vi "Sequence.Test.Unload.vi"(7 "Code in":T1={"Ready"=FALSE, "DoubleOrder"=FALSE, "OrderDone"=FALSE, "AllowSingleSlot"=FALSE, "TunedA"=FALSE, "TunedB"=FALSE, "CheckDM"=FALSE, "ThresholdA"=0, "ThresholdB"=0, "Plate"=enum."Wabco", "ImgPath"=path "", "Variant"={"State"=enum."Init", "ImgPath"=path "", "WabcoPlate"="", "WabcoProduct"="", "ClientProduct"="", "ClientPlate"="", "TotalQuantity"=0, "OrderQuantity"=0, "Serial"=0, "Wabco"={"LaserJob"="", "AdditionalTxt"="037", "FactoryCode"="", "RevID"=0, "ForkID"=0, "FailuresLimit"=0, "GlobalCnt"=0, "Bank"=0, "SerialFormat"=enum."6 dig", "CoordA"={"X"=0.0, "Y"=0.0, "Angle"=0.0}, "CoordB"={"X"=0.0, "Y"=0.0, "Angle"=0.0}, "DMCconfig"=0}, "Client"={"LaserJob"="", "AdditionalTxt"="", "FactoryCode"="037", "RevID"=0, "ForkID"=0, "FailuresLimit"=0, "GlobalCnt"=0, "Bank"=0, "SerialFormat"=enum."6 dig", "CoordA"={"X"=0.0, "Y"=0.0, "Angle"=0.0}, "CoordB"={"X"=0.0, "Y"=0.0, "Angle"=0.0}, "DMCconfig"=0}}}, 8 "error in":errorcluster, 11 "Data in":T8) -> (0 "error out":errorcluster, 3 "Data out":T8)   [LabVIEW 2016]
uses:
  Sequence.Test.Status.ctl
  Sequence.Slot.StatusData.ctl
  Sequence.Test.Unload.Status.ctl
  Sequence.Prod.StatusData.ctl
  Sequence.Step.Status.ctl
  Sequence.Test.BreakReason.ctl
  Sequence.Code.Sets.ctl
  Sequence.PlateType.ctl
  Logger/Logger.Variant.Sets.ctl
  Station/Station.Changeover.State.vi
  Station/Station.Plate.Properties.ctl
  Sequence.Code.SerialFormat.ctl
  Drivers/V7310/LowLevel/V7310.Job.Sets.ctl
  Drivers/FestoCPX/Station/FestoCPX.Station.ProdArmPosition.ctl
  Station/Station.ProductSlot.ctl
  Station/Station.ValvePosition.ctl
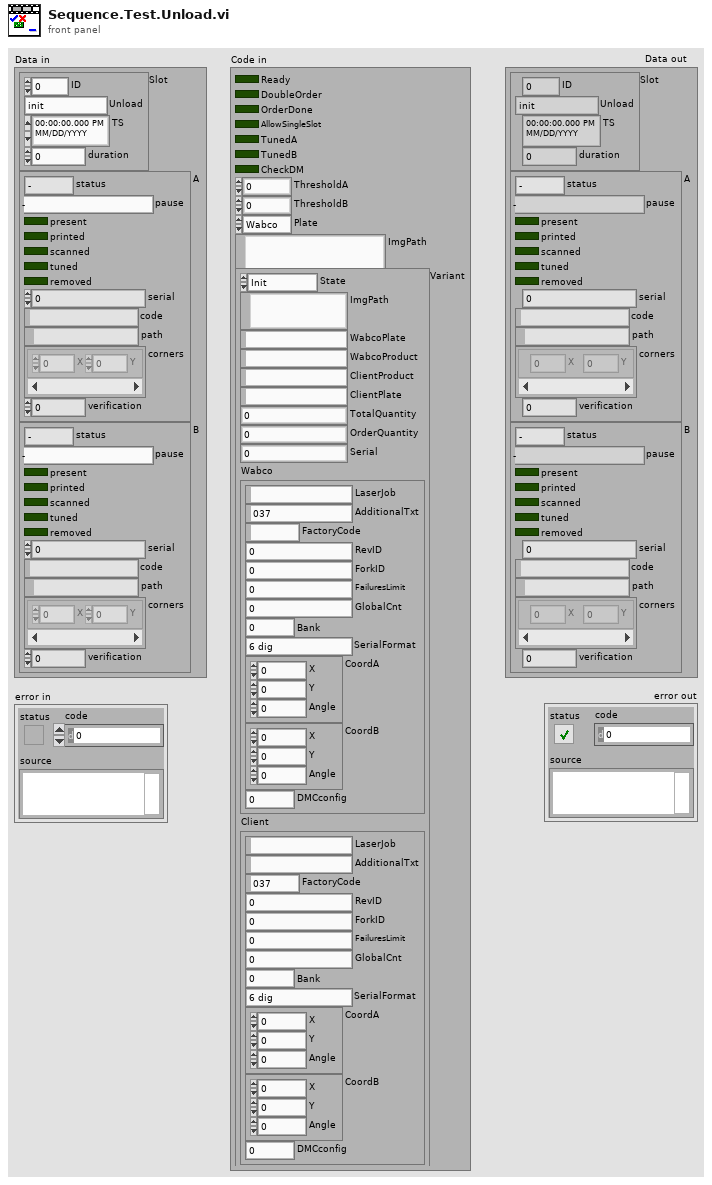
[diagram p1: front panel]
types:
  T1 = typedef "Sequence.Code.Sets.ctl" = cluster{"Ready":bool, "DoubleOrder":bool, "OrderDone":bool, "AllowSingleSlot":bool, "TunedA":bool, "TunedB":bool, "CheckDM":bool, "ThresholdA":u8, "ThresholdB":u8, "Plate":T2, "ImgPath":path, "Variant":T3}
  T2 = typedef "Sequence.PlateType.ctl" = enum16{"Wabco", "Client"}
  T3 = typedef "Logger.Variant.Sets.ctl" = cluster{"State":T4, "ImgPath":path, "WabcoPlate":string, "WabcoProduct":string, "ClientProduct":string, "ClientPlate":string, "TotalQuantity":u16, "OrderQuantity":u16, "Serial":i32, "Wabco":T5, "Client":T5}
  T4 = typedef "Station.Changeover.State.vi" = enum16{"Init", "Scaning", "NOK", "Wait for ack", "Ready"}
  T5 = typedef "Station.Plate.Properties.ctl" = cluster{"LaserJob":string, "AdditionalTxt":string, "FactoryCode":string, "RevID":u8, "ForkID":u8, "FailuresLimit":u16, "GlobalCnt":i32, "Bank":u8, "SerialFormat":T6, "CoordA":T7, "CoordB":T7, "DMCconfig":i32}
  T6 = typedef "Sequence.Code.SerialFormat.ctl" = enum8{"", "6 dig", "7 dig"}
  T7 = typedef "V7310.Job.Sets.ctl" = cluster{"X":dbl, "Y":dbl, "Angle":dbl}
  T8 = typedef "Sequence.Test.Status.ctl" = cluster{"Slot":T9, "A":T11, "B":T11}
  T9 = typedef "Sequence.Slot.StatusData.ctl" = cluster{"ID":i32, "Unload":T10, "TS":timestamp, "duration":u32}
  T10 = typedef "Sequence.Test.Unload.Status.ctl" = enum16{"init", "check NOK", "check OK", "wait on NOK", "wait on OK", "wait on Unload", "done"}
  T11 = typedef "Sequence.Prod.StatusData.ctl" = cluster{"status":T12, "pause":T13, "present":bool, "printed":bool, "scanned":bool, "tuned":bool, "removed":bool, "serial":i32, "code":string, "path":path, "corners":cluster{"X":i32, "Y":i32}[], "verification":u8}
  T12 = typedef "Sequence.Step.Status.ctl" = enum16{"-", "Pending", "Running", "Skipped", "Passed", "Failed", "Done", "Error", "Aborted", "Stopped"}
  T13 = typedef "Sequence.Test.BreakReason.ctl" = enum16{"-", "NOK container", "OK container", "Rev empty", "Rev missing", "Rev wrong", "Fork missing", "Fork wrong", "NOK limit", "Unload failure", "Single slot", "Part done", "Err: Prod move work", "Err: Prod move home", "Err: Prod lift work", "Err: Prod lift home", "Err: Prod Arm Work", "Err: Prod Arm NOK", "Err: Prod Arm OK", "Err: Prod NOK suck", "Err: Prod NOK drop", "Err: Prod OK missing", "Err: Prod OK suck", "Err: Prod OK drop"}
  T14 = typedef "FestoCPX.Station.ProdArmPosition.ctl" = enum16{"Work", "OK", "NOK"}
  T15 = typedef "Station.ProductSlot.ctl" = enum8{"A", "B"}
  T16 = typedef "FestoCPX.Station.ProdPresent.ctl" = cluster{"Slot1":cluster{"A":bool, "B":bool}, "Slot2":cluster{"A":bool, "B":bool}, "Slot3":cluster{"A":bool, "B":bool}, "Slot4":cluster{"A":bool, "B":bool}, "Final":cluster{"A":bool, "B":bool}, "OK":cluster{"A":bool, "B":bool}, "Container":cluster{"OK":bool, "NOK":bool}}
  T17 = typedef "Station.ValvePosition.ctl" = enum16{"Home", "Work"}
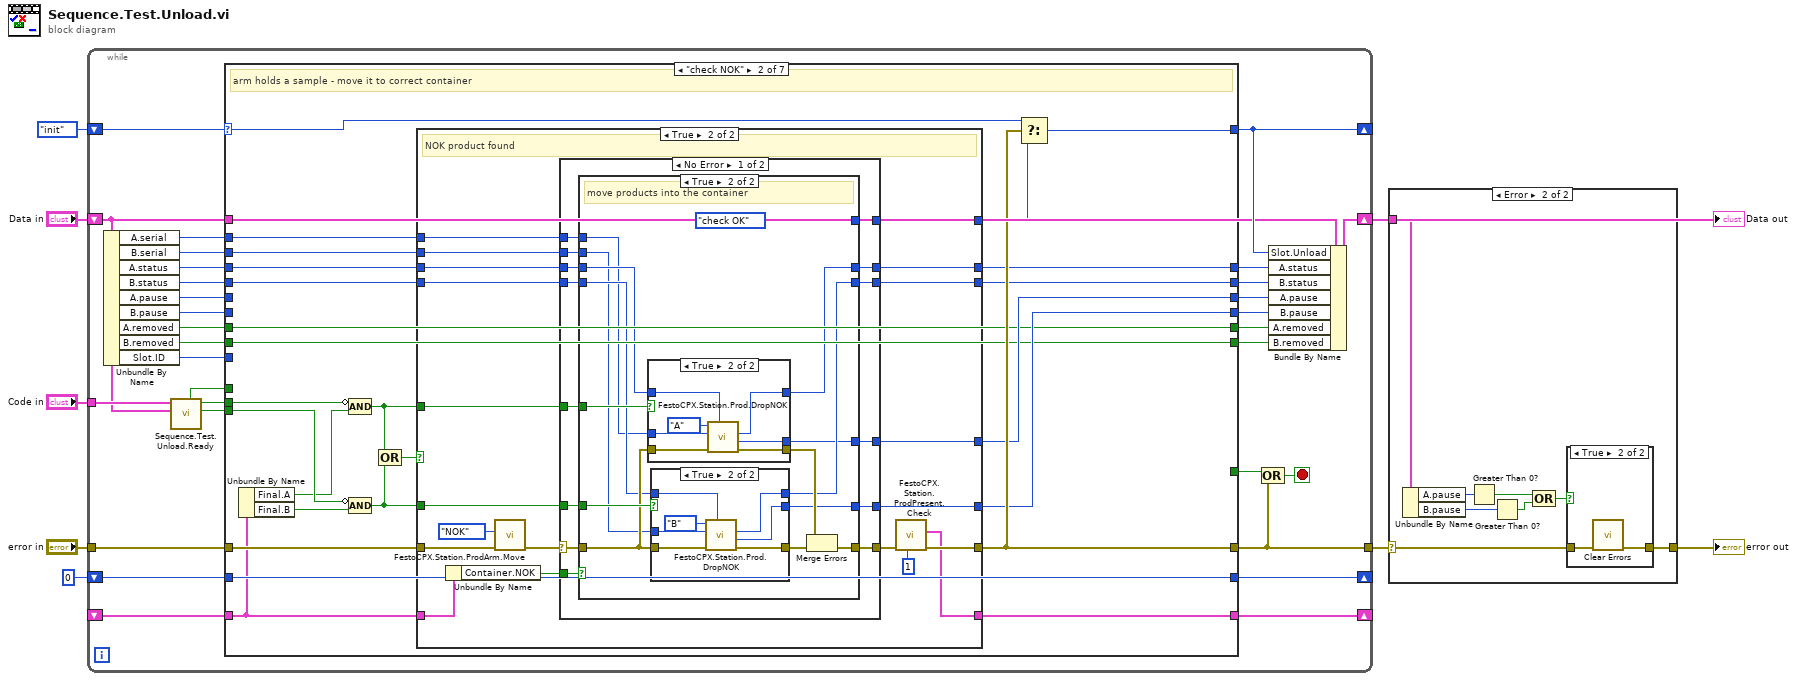
[diagram p0: block diagram]
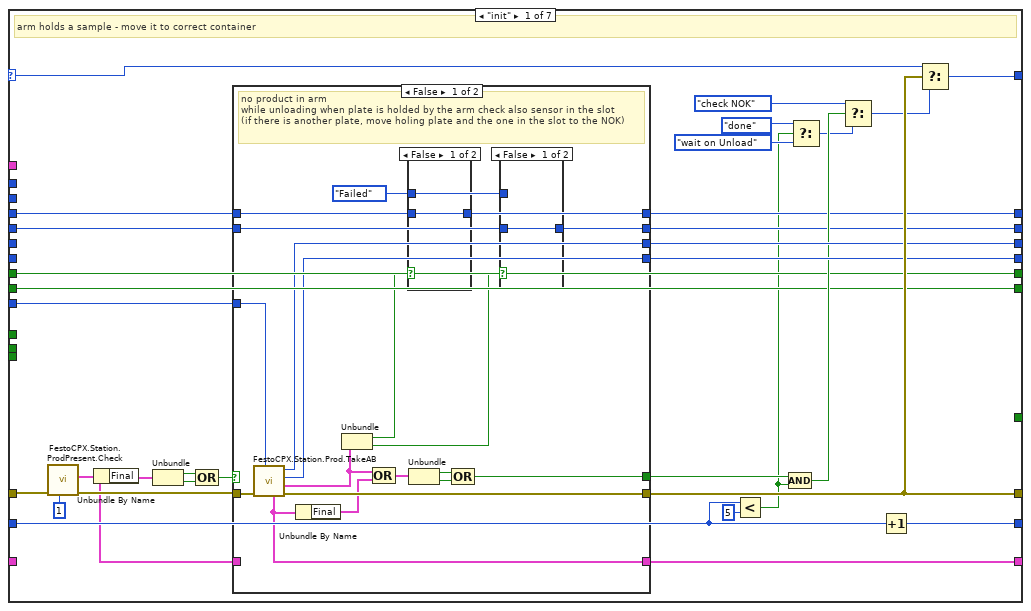
[diagram p2: hidden frame]
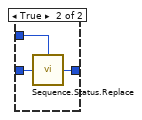
[diagram p3: hidden frame]
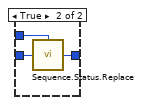
[diagram p4: hidden frame]
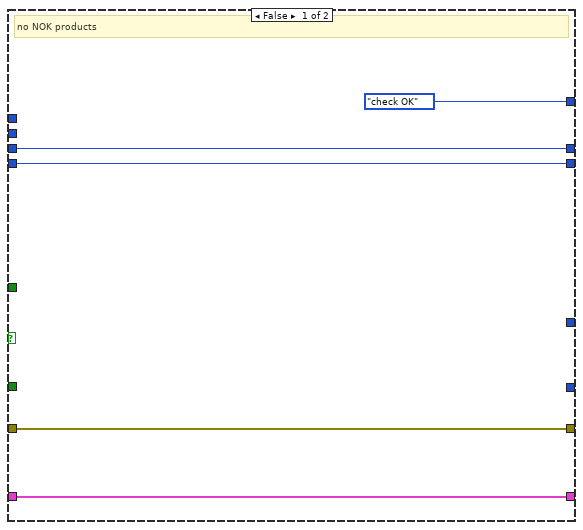
[diagram p6: hidden frame]
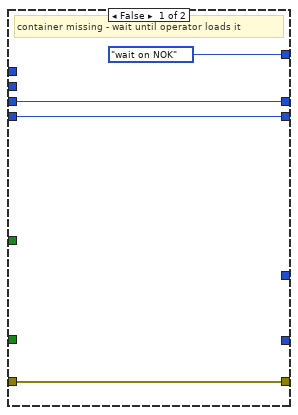
[diagram p7: hidden frame]
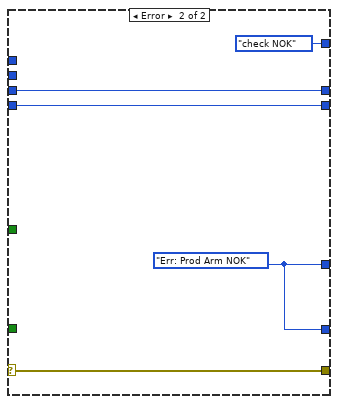
[diagram p10: hidden frame]
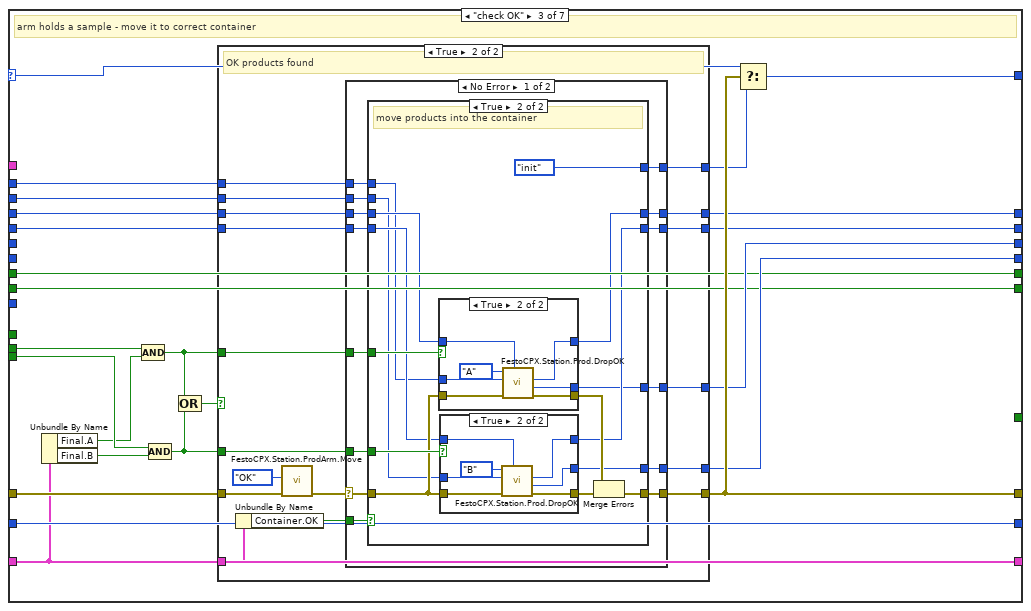
[diagram p11: hidden frame]
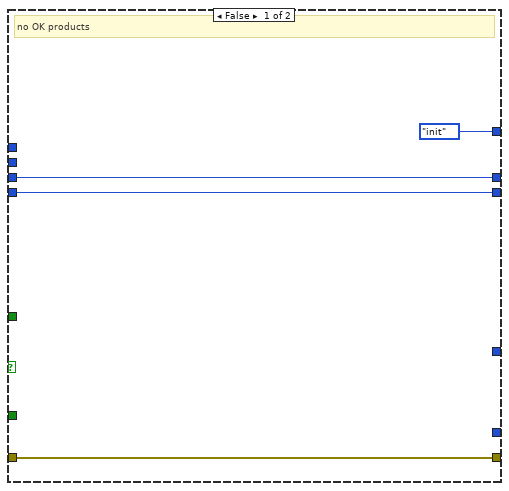
[diagram p12: hidden frame]
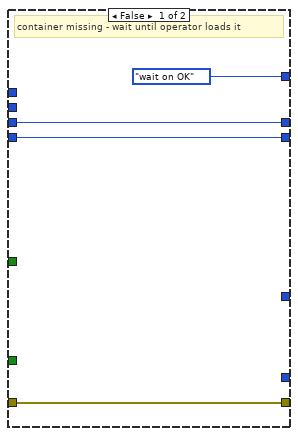
[diagram p13: hidden frame]
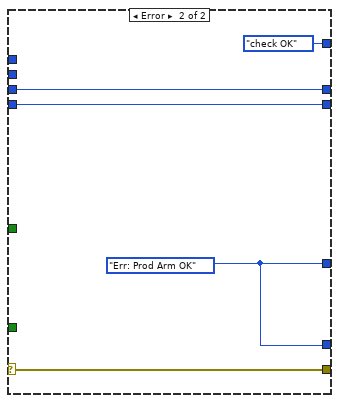
[diagram p16: hidden frame]
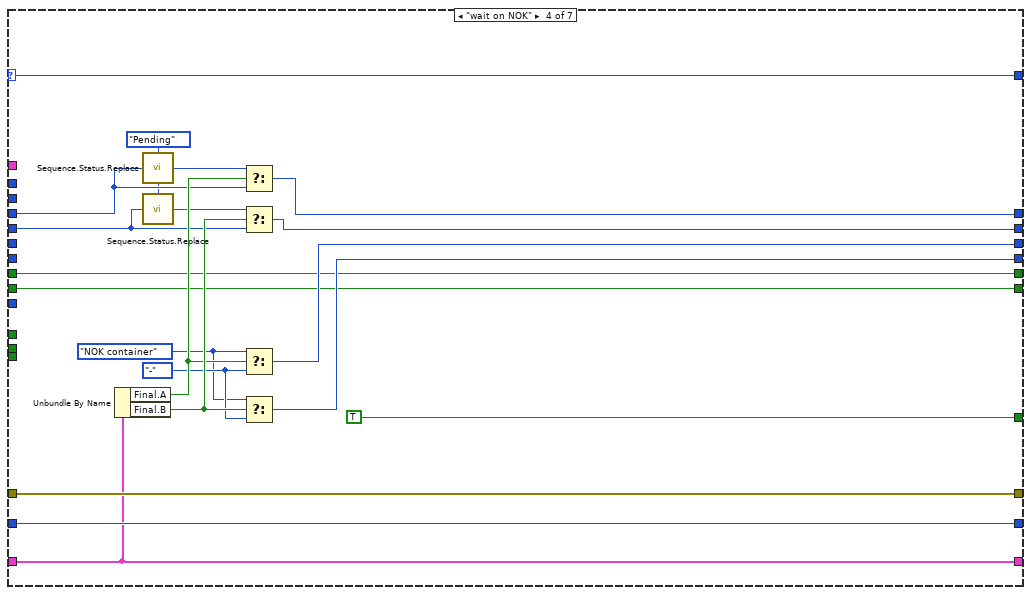
[diagram p17: hidden frame]
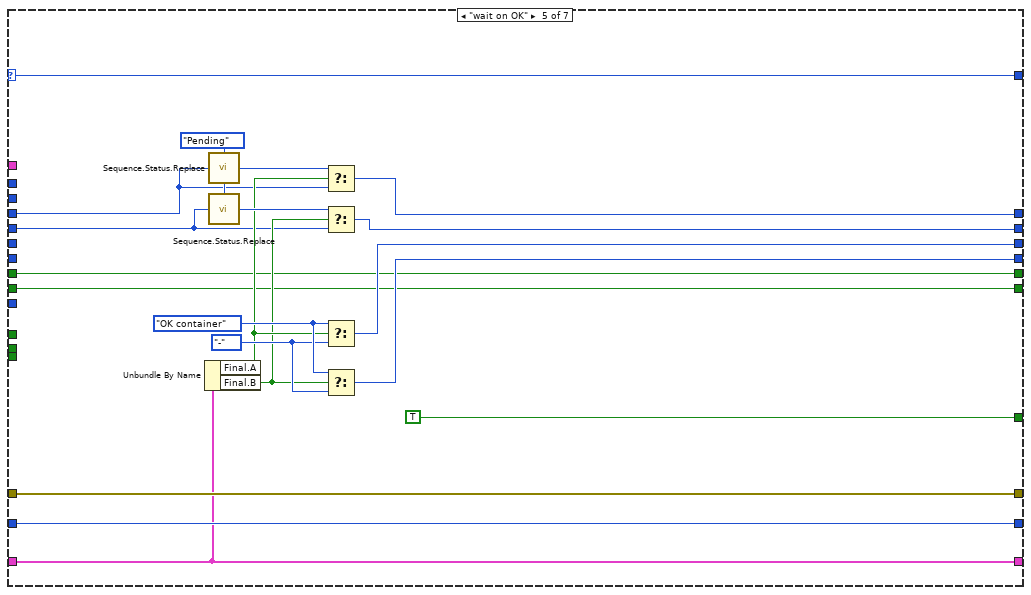
[diagram p18: hidden frame]
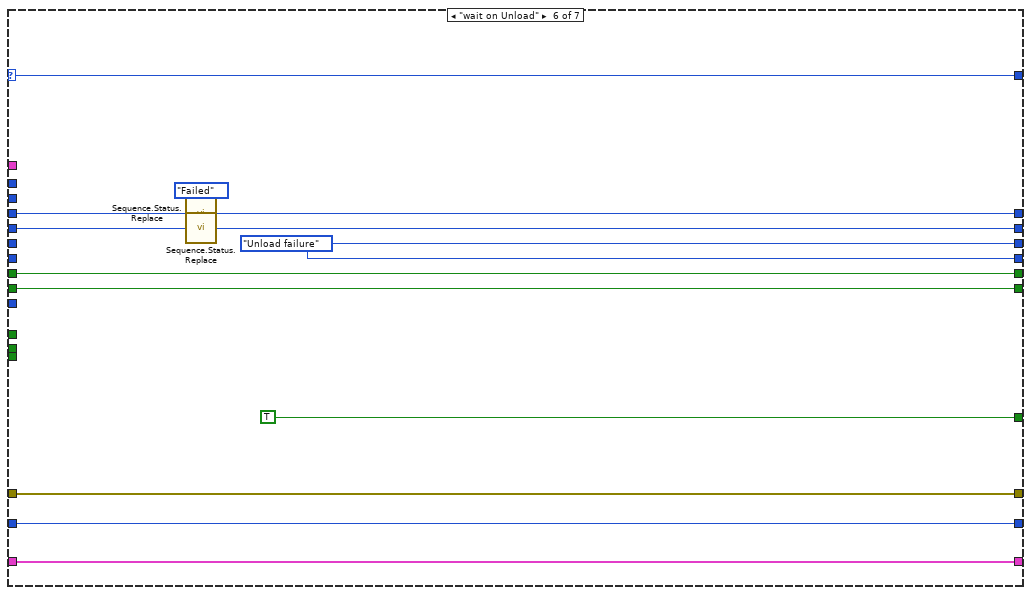
[diagram p19: hidden frame]
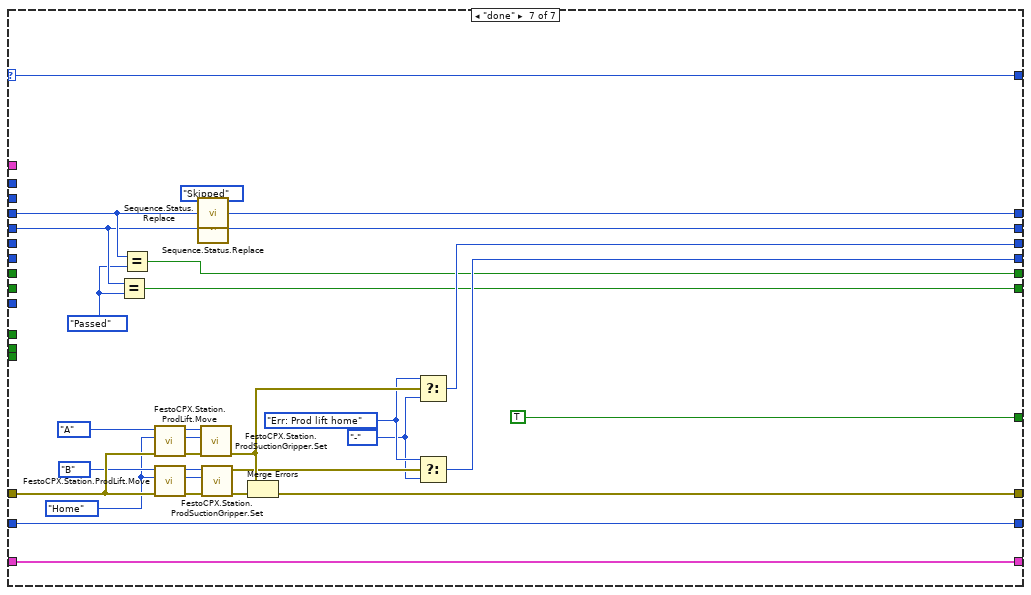
[diagram p20: hidden frame]
diagram:
  n1 = while {
    shift-right: [w34] -> w1
    shift-left: "Data in" -> [w25]
    tunnel: "error in" -> [w15]
    tunnel: [w37] -> w3
    shift-right: [w33] -> _
    shift-left: Sequence.Test.Unload.Status."init" ("Slot.Unload") -> [w36]
    tunnel: "Code in" -> [w26]
    shift-right: [w21] -> _
    shift-left: 0 -> [w22]
    shift-right: [w14] -> _
    shift-left: _ -> [w13]
    stop <- w39 stop-if-true
    n2 = Unbundle By Name(w25) -> ("A.serial"=w28:i32, "B.serial"=w27:i32, "A.status"=w31:T12, "B.status"=w32:T12, "A.pause"=w18:T13, "B.pause"=w17:T13, "A.removed"=w12:bool, "B.removed"=w11:bool, "Slot.ID"=w35:i32)
    n3 = call "Sequence.Test.Unload.Ready.vi"("Data in"=w25, "Code"=w26) -> ("OK B"=w23:bool, "OK A"=w24:bool, "PartialOrder"=w16:bool)  [unwired: 7 in]
    n4 = case shown="\"check NOK\"" w36 {
      selector: w36 -> [w66 w121 w227 w330 w350 w363 w382]
      tunnel: w15 -> [w55 w125 w216 w328 w348 w361 w387]
      tunnel: [w71 w128 w233 w328 w348 w361 w381] -> w37
      tunnel: [_ _ _ TRUE TRUE TRUE TRUE] -> w38
      tunnel: [w70 w126 w231 w330 w350 w363 w382] -> w33
      tunnel: w35 -> [w51 _ _ _ _ _ _]
      tunnel: w25 -> [_ _ _ _ _ _ _]
      tunnel: w32 -> [w47 w118 w223 w316 w337 w356 w366]
      tunnel: w31 -> [w49 w120 w224 w315 w336 w359 w368]
      tunnel: [w46 w117 w226 w322 w335 w357 w379] -> w30
      tunnel: [w48 w119 w225 w323 w334 w358 w380] -> w29
      tunnel: [w64 w113 w217 w327 w347 w354 w371] -> w20
      tunnel: [w63 w112 w212 w326 w346 w354 w370] -> w19
      tunnel: w28 -> [_ w116 w222 _ _ _ _]
      tunnel: w27 -> [_ w115 w221 _ _ _ _]
      tunnel: w24 -> [_ w111 w219 _ _ _ _]
      tunnel: w23 -> [_ w110 w220 _ _ _ _]
      tunnel: w22 -> [w58 w114 w218 w321 w345 w360 w377]
      tunnel: [w65 w114 w218 w321 w345 w360 w377] -> w21
      tunnel: w18 -> [_ _ _ _ _ _ _]
      tunnel: w17 -> [_ _ _ _ _ _ _]
      tunnel: w16 -> [_ _ _ _ _ _ _]
      tunnel: [w62 w109 w213 w313 w333 w353 w369] -> w14
      tunnel: w13 -> [_ w108 w213 w313 w333 w353 w369]
      tunnel: w12 -> [w45 w105 w211 w312 w332 w352 _]
      tunnel: w11 -> [w44 w104 w210 w311 w331 w351 _]
      tunnel: [w45 w105 w211 w312 w332 w352 w367] -> w10
      tunnel: [w44 w104 w210 w311 w331 w351 w364] -> w9
      frame "init" {
        # "arm holds a sample - move it to correct container"
        n5 = call "FestoCPX.Station.ProdPresent.Check.vi"("Stab Counter (0)"=1 ("Max Stab time [ms] (0)"), "error in"=w55) -> ("error out"=w54:errorcluster, "Prod Present"=w52:T16)  [unwired: 4 in, 4 out]
        n6 = Unbundle By Name(w52) -> ("Final"=w53:cluster{"A":bool, "B":bool})
        n7 = Unbundle(w53) -> ("A"=w69:bool, "B"=w68:bool)
        n8 = Compound Arithmetic op=OR(w69, w68) -> (w67:bool)
        n9 = case shown="False" w67 {
          selector: w67 -> [_ w101]
          tunnel: [w80 w103] -> w71
          tunnel: w54 -> [w90 w103]
          tunnel: [w89 _] -> w64
          tunnel: [w88 _] -> w63
          tunnel: [w79 w102] -> w62
          tunnel: w52 -> [_ w102]
          tunnel: [w75 w101] -> w57
          tunnel: w51 -> [w87 _]
          tunnel: w49 -> [w86 w100]
          tunnel: [w83 w100] -> w48
          tunnel: w47 -> [w84 w99]
          tunnel: [w82 w99] -> w46
          frame False {
            w85 = Sequence.Step.Status."Failed" ("t")
            # "no product in arm\nwhile unloading when plate is holded by the arm check also sensor in the slot \n(if there is another plate, move holing plate and the one in the slot to the NOK)"
            n10 = call "FestoCPX.Station.Prod.TakeAB.vi"("SuckerID"=w87, "error in"=w90) -> ("error out"=w80:errorcluster, "Slot"=w73:cluster{"A":bool, "B":bool}, "Error reason B"=w88:T13, "Error reason A"=w89:T13, "Prod Present"=w79:T16)  [unwired: 5 in]
            n11 = Unbundle By Name(w79) -> ("Final"=w72:cluster{"A":bool, "B":bool})
            n12 = Unbundle(w73) -> ("A"=w74:bool, "B"=w81:bool)
            n13 = Compound Arithmetic op=OR(w73, w72) -> (w78:cluster{"A":bool, "B":bool})
            n14 = case shown="False" w74 {
              tunnel: w86 -> [w95 w98]
              tunnel: w85 -> [_ w97]
              tunnel: [w95 w96] -> w83
              frame False {
              }
              frame True {
                n15 = call "Sequence.Status.Replace.vi"("old status"=w98, "new status (Done)"=w97) -> ("status out"=w96:T12)
              }
            }
            n16 = Unbundle(w78) -> ("A"=w77:bool, "B"=w76:bool)
            n17 = Compound Arithmetic op=OR(w77, w76) -> (w75:bool)
            n18 = case shown="False" w81 {
              tunnel: w84 -> [w91 w94]
              tunnel: w85 -> [_ w93]
              tunnel: [w91 w92] -> w82
              frame False {
              }
              frame True {
                n19 = call "Sequence.Status.Replace.vi"("old status"=w94, "new status (Done)"=w93) -> ("status out"=w92:T12)
              }
            }
          }
          frame True {
            # "arm already holds product"
          }
        }
        n20 = Less?(x=w58, y=5) -> (x < y?=w41:bool)
        n21 = Compound Arithmetic op=AND(w57, w41) -> (w56:bool)
        n22 = Select(t=Sequence.Test.Unload.Status."done" ("Slot.Unload"), s=w41, f=Sequence.Test.Unload.Status."wait on Unload" ("Slot.Unload")) -> (s? t:f=w40:T10)
        n23 = Select(t=Sequence.Test.Unload.Status."check NOK" ("Slot.Unload"), s=w56, f=w40) -> (s? t:f=w59:T10)
        n24 = Increment(x=w58) -> (x+1=w65:i32)
        n25 = Select(t=w66, s=w71, f=w59) -> (s? t:f=w70:T10)
      }
      frame "check NOK" {
        # "arm holds a sample - move it to correct container"
        n26 = Unbundle By Name(w108) -> ("Final.A"=w107:bool, "Final.B"=w106:bool)
        n27 = Compound Arithmetic op=AND(invert w111, w107) -> (w123:bool)
        n28 = Compound Arithmetic op=AND(invert w110, w106) -> (w122:bool)
        n29 = Compound Arithmetic op=OR(w123, w122) -> (w124:bool)
        n30 = case shown="True" w124 {
          tunnel: w123 -> [_ w153]
          tunnel: w122 -> [_ w152]
          tunnel: w125 -> [w132 w150]
          tunnel: [w132 w136] -> w128
          tunnel: [Sequence.Test.Unload.Status."check OK" ("Slot.Unload") w149] -> w127
          tunnel: w120 -> [w131 w148]
          tunnel: [w131 w147] -> w119
          tunnel: w118 -> [w130 w146]
          tunnel: [w130 w145] -> w117
          tunnel: w116 -> [_ w144]
          tunnel: w115 -> [_ w143]
          tunnel: [_ w141] -> w113
          tunnel: [_ w140] -> w112
          tunnel: [w129 w135] -> w109
          tunnel: w108 -> [w129 w139]
          frame False {
            # "no NOK products"
          }
          frame True {
            # "NOK product found"
            n31 = Unbundle By Name(w139) -> ("Container.NOK"=w142:bool)
            n32 = call "FestoCPX.Station.ProdArm.Move.vi"("error in"=w150, "Product Status"=FestoCPX.Station.ProdArmPosition."NOK") -> ("error out"=w138:errorcluster)  [unwired: 9 in]
            n33 = case shown="No Error" w138 {
              selector: w138 -> [w154 w209]
              tunnel: w153 -> [w167 _]
              tunnel: w152 -> [w166 _]
              tunnel: [w165 w209] -> w137
              tunnel: [w164 Sequence.Test.Unload.Status."check NOK" ("Slot.Unload")] -> w149
              tunnel: w148 -> [w163 w208]
              tunnel: [w162 w208] -> w147
              tunnel: w146 -> [w161 w207]
              tunnel: [w160 w207] -> w145
              tunnel: w144 -> [w159 _]
              tunnel: w143 -> [w158 _]
              tunnel: w142 -> [w157 _]
              tunnel: [w156 w206] -> w141
              tunnel: [w155 w206] -> w140
              frame No Error {
                n34 = case shown="True" w157 {
                  tunnel: w167 -> [_ w186]
                  tunnel: w166 -> [_ w185]
                  tunnel: [w170 w182] -> w165
                  tunnel: w154 -> [w170 w181]
                  tunnel: [Sequence.Test.Unload.Status."wait on NOK" ("Slot.Unload") Sequence.Test.Unload.Status."check OK" ("Slot.Unload")] -> w164
                  tunnel: [w169 w178] -> w162
                  tunnel: w163 -> [w169 w179]
                  tunnel: w161 -> [w168 w176]
                  tunnel: [w168 w177] -> w160
                  tunnel: w159 -> [_ w175]
                  tunnel: w158 -> [_ w174]
                  tunnel: [_ w173] -> w156
                  tunnel: [_ w172] -> w155
                  frame False {
                    # "container missing - wait until operator loads it"
                  }
                  frame True {
                    # "move products into the container"
                    n35 = case shown="True" w186 {
                      tunnel: w181 -> [w197 w204]
                      tunnel: [w197 w203] -> w183
                      tunnel: w179 -> [w196 w198]
                      tunnel: [w196 w200] -> w178
                      tunnel: w175 -> [_ w201]
                      tunnel: [_ w199] -> w173
                      frame False {
                      }
                      frame True {
                        n36 = call "FestoCPX.Station.Prod.DropNOK.vi"("prev status"=w198, "error in"=w204, "Serial"=w201, "Slot"=Station.ProductSlot."A") -> ("error out"=w203:errorcluster, "Pause status"=w199:T13, "Final status"=w200:T12)  [unwired: 5 in]
                      }
                    }
                    n37 = case shown="True" w185 {
                      tunnel: w181 -> [w188 w194]
                      tunnel: [w188 w193] -> w184
                      tunnel: [w187 w191] -> w177
                      tunnel: w176 -> [w187 w189]
                      tunnel: w174 -> [_ w192]
                      tunnel: [_ w190] -> w172
                      frame False {
                      }
                      frame True {
                        n38 = call "FestoCPX.Station.Prod.DropNOK.vi"("prev status"=w189, "error in"=w194, "Serial"=w192, "Slot"=Station.ProductSlot."B") -> ("error out"=w193:errorcluster, "Pause status"=w190:T13, "Final status"=w191:T12)  [unwired: 5 in]
                      }
                    }
                    n39 = Merge Errors(w183, w184) -> (w182:errorcluster)
                  }
                }
              }
              frame Error {
                w206 = Sequence.Test.BreakReason."Err: Prod Arm NOK" ("A.pause")
              }
            }
            n40 = call "FestoCPX.Station.ProdPresent.Check.vi"("Stab Counter (0)"=1 ("Max Stab time [ms] (0)"), "error in"=w137) -> ("error out"=w136:errorcluster, "Prod Present"=w135:T16)  [unwired: 4 in, 4 out]
          }
        }
        n41 = Select(t=w121, s=w128, f=w127) -> (s? t:f=w126:T10)
      }
      frame "check OK" {
        # "arm holds a sample - move it to correct container"
        n42 = Unbundle By Name(w213) -> ("Final.A"=w214:bool, "Final.B"=w215:bool)
        n43 = Compound Arithmetic op=AND(w219, w214) -> (w229:bool)
        n44 = Compound Arithmetic op=AND(w220, w215) -> (w228:bool)
        n45 = Compound Arithmetic op=OR(w229, w228) -> (w230:bool)
        n46 = case shown="True" w230 {
          tunnel: w229 -> [_ w242]
          tunnel: w228 -> [_ w241]
          tunnel: w216 -> [w236 w252]
          tunnel: [w236 w253] -> w233
          tunnel: [Sequence.Test.Unload.Status."init" ("Slot.Unload") w251] -> w232
          tunnel: w223 -> [w235 w250]
          tunnel: w224 -> [w234 w249]
          tunnel: [w235 w248] -> w226
          tunnel: [w234 w247] -> w225
          tunnel: w222 -> [_ w246]
          tunnel: w221 -> [_ w245]
          tunnel: [_ w244] -> w217
          tunnel: [_ w243] -> w212
          tunnel: w213 -> [_ w240]
          frame False {
            # "no OK products"
          }
          frame True {
            # "OK products found"
            n47 = Unbundle By Name(w240) -> ("Container.OK"=w239:bool)
            n48 = call "FestoCPX.Station.ProdArm.Move.vi"("error in"=w252, "Product Status"=FestoCPX.Station.ProdArmPosition."OK") -> ("error out"=w238:errorcluster)  [unwired: 9 in]
            n49 = case shown="No Error" w238 {
              selector: w238 -> [w255 w307]
              tunnel: [w268 w307] -> w253
              tunnel: w239 -> [w267 _]
              tunnel: [w266 Sequence.Test.Unload.Status."check OK" ("Slot.Unload")] -> w251
              tunnel: w250 -> [w265 w308]
              tunnel: w249 -> [w264 w309]
              tunnel: [w263 w308] -> w248
              tunnel: [w262 w309] -> w247
              tunnel: w246 -> [w261 _]
              tunnel: w245 -> [w260 _]
              tunnel: [w259 w306] -> w244
              tunnel: [w258 w306] -> w243
              tunnel: w242 -> [w257 _]
              tunnel: w241 -> [w256 _]
              frame No Error {
                n50 = case shown="True" w267 {
                  tunnel: w257 -> [_ w287]
                  tunnel: w256 -> [_ w286]
                  tunnel: [w271 w283] -> w268
                  tunnel: w255 -> [w271 w282]
                  tunnel: [Sequence.Test.Unload.Status."wait on OK" ("Slot.Unload") Sequence.Test.Unload.Status."init" ("Slot.Unload")] -> w266
                  tunnel: [w270 w280] -> w262
                  tunnel: w265 -> [w269 w277]
                  tunnel: w264 -> [w270 w278]
                  tunnel: [w269 w279] -> w263
                  tunnel: w261 -> [_ w276]
                  tunnel: w260 -> [_ w275]
                  tunnel: [_ w274] -> w259
                  tunnel: [_ w273] -> w258
                  frame False {
                    # "container missing - wait until operator loads it"
                  }
                  frame True {
                    # "move products into the container"
                    n51 = case shown="True" w287 {
                      tunnel: w282 -> [w298 w305]
                      tunnel: [w298 w303] -> w284
                      tunnel: [w297 w301] -> w280
                      tunnel: w278 -> [w297 w299]
                      tunnel: w276 -> [_ w302]
                      tunnel: [_ w300] -> w274
                      frame False {
                      }
                      frame True {
                        n52 = call "FestoCPX.Station.Prod.DropOK.vi"("prev status"=w299, "error in"=w305, "Serial"=w302, "Slot"=Station.ProductSlot."A") -> ("error out"=w303:errorcluster, "Pause status"=w300:T13, "Final status"=w301:T12)  [unwired: 5 in]
                      }
                    }
                    n53 = case shown="True" w286 {
                      tunnel: w282 -> [w289 w295]
                      tunnel: [w289 w294] -> w285
                      tunnel: [w288 w292] -> w279
                      tunnel: w277 -> [w288 w290]
                      tunnel: w275 -> [_ w293]
                      tunnel: [_ w291] -> w273
                      frame False {
                      }
                      frame True {
                        n54 = call "FestoCPX.Station.Prod.DropOK.vi"("prev status"=w290, "error in"=w295, "Serial"=w293, "Slot"=Station.ProductSlot."B") -> ("error out"=w294:errorcluster, "Pause status"=w291:T13, "Final status"=w292:T12)  [unwired: 5 in]
                      }
                    }
                    n55 = Merge Errors(w284, w285) -> (w283:errorcluster)
                  }
                }
              }
              frame Error {
                w306 = Sequence.Test.BreakReason."Err: Prod Arm OK" ("A.pause")
              }
            }
          }
        }
        n56 = Select(t=w227, s=w233, f=w232) -> (s? t:f=w231:T10)
      }
      frame "wait on NOK" {
        w319 = Sequence.Test.BreakReason."NOK container" ("A.pause")
        w320 = Sequence.Test.BreakReason."-" ("A.pause")
        w314 = Sequence.Step.Status."Pending" ("t")
        n57 = Unbundle By Name(w313) -> ("Final.A"=w324:bool, "Final.B"=w325:bool)
        n58 = call "Sequence.Status.Replace.vi"("old status"=w315, "new status (Done)"=w314) -> ("status out"=w318:T12)
        n59 = call "Sequence.Status.Replace.vi"("old status"=w316, "new status (Done)"=w314) -> ("status out"=w317:T12)
        n60 = Select(t=w318, s=w324, f=w315) -> (s? t:f=w323:T12)
        n61 = Select(t=w317, s=w325, f=w316) -> (s? t:f=w322:T12)
        n62 = Select(t=w319, s=w324, f=w320) -> (s? t:f=w327:T13)
        n63 = Select(t=w319, s=w325, f=w320) -> (s? t:f=w326:T13)
      }
      frame "wait on OK" {
        w340 = Sequence.Step.Status."Pending" ("t")
        w344 = Sequence.Test.BreakReason."OK container" ("A.pause")
        w343 = Sequence.Test.BreakReason."-" ("A.pause")
        n64 = Unbundle By Name(w333) -> ("Final.A"=w339:bool, "Final.B"=w338:bool)
        n65 = call "Sequence.Status.Replace.vi"("old status"=w336, "new status (Done)"=w340) -> ("status out"=w342:T12)
        n66 = call "Sequence.Status.Replace.vi"("old status"=w337, "new status (Done)"=w340) -> ("status out"=w341:T12)
        n67 = Select(t=w342, s=w339, f=w336) -> (s? t:f=w334:T12)
        n68 = Select(t=w341, s=w338, f=w337) -> (s? t:f=w335:T12)
        n69 = Select(t=w344, s=w339, f=w343) -> (s? t:f=w347:T13)
        n70 = Select(t=w344, s=w338, f=w343) -> (s? t:f=w346:T13)
      }
      frame "wait on Unload" {
        w354 = Sequence.Test.BreakReason."Unload failure" ("A.pause")
        w355 = Sequence.Step.Status."Failed" ("t")
        n71 = call "Sequence.Status.Replace.vi"("old status"=w359, "new status (Done)"=w355) -> ("status out"=w358:T12)
        n72 = call "Sequence.Status.Replace.vi"("old status"=w356, "new status (Done)"=w355) -> ("status out"=w357:T12)
      }
      frame "done" {
        w365 = Sequence.Step.Status."Passed" ("y")
        w372 = Sequence.Test.BreakReason."-" ("Pause status")
        w373 = Sequence.Test.BreakReason."Err: Prod lift home" ("Pause status")
        w378 = Sequence.Step.Status."Skipped" ("new status (Done)")
        w384 = Station.ProductSlot."B" ("Slot")
        w383 = Station.ValvePosition."Home" ("Position")
        w386 = Station.ProductSlot."A" ("Slot")
        n73 = Equal?(x=w366, y=w365) -> (x = y?=w364:bool)
        n74 = Equal?(x=w368, y=w365) -> (x = y?=w367:bool)
        n75 = call "FestoCPX.Station.ProdLift.Move.vi"("error in"=w387, "Position"=w383, "Slot"=w386) -> ("error out"=w376:errorcluster)  [unwired: 8 in]
        n76 = call "FestoCPX.Station.ProdLift.Move.vi"("error in"=w387, "Position"=w383, "Slot"=w384) -> ("error out"=w385:errorcluster)  [unwired: 8 in]
        n77 = call "Sequence.Status.Replace.vi"("old status"=w368, "new status (Done)"=w378) -> ("status out"=w380:T12)
        n78 = call "Sequence.Status.Replace.vi"("old status"=w366, "new status (Done)"=w378) -> ("status out"=w379:T12)
        n79 = call "FestoCPX.Station.ProdSuctionGripper.Set.vi"("error in"=w376, "Position"=w383, "Slot"=w386) -> ("error out"=w375:errorcluster)  [unwired: 7 in, 1 out]
        n80 = call "FestoCPX.Station.ProdSuctionGripper.Set.vi"("error in"=w385, "Position"=w383, "Slot"=w384) -> ("error out"=w374:errorcluster)  [unwired: 7 in, 1 out]
        n81 = Merge Errors(w375, w374) -> (w381:errorcluster)
        n82 = Select(t=w373, s=w375, f=w372) -> (s? t:f=w371:T13)
        n83 = Select(t=w373, s=w374, f=w372) -> (s? t:f=w370:T13)
      }
    }
    n84 = Compound Arithmetic op=OR(w38, w37) -> (w39:bool)
    n85 = Bundle By Name(cluster=w25, "Slot.Unload"=w33, "A.status"=w29, "B.status"=w30, "A.pause"=w20, "B.pause"=w19, "A.removed"=w10, "B.removed"=w9) -> (w34:T8)
  }
  "Data out" <- w1
  n86 = case shown="Error" w3 {
    selector: w3 -> [w389 w397]
    tunnel: w1 -> [_ w391]
    tunnel: [w389 w396] -> w2
    frame No Error {
    }
    frame Error {
      n87 = Unbundle By Name(w391) -> ("A.pause"=w394:T13, "B.pause"=w393:T13)
      n88 = Greater Than 0?(x=w394) -> (x > 0?=w395:bool)
      n89 = Greater Than 0?(x=w393) -> (x > 0?=w390:bool)
      n90 = Compound Arithmetic op=OR(w395, w390) -> (w392:bool)
      n91 = case shown="True" w392 {
        tunnel: w397 -> [w398 w400]
        tunnel: [w398 w399] -> w396
        frame False {
        }
        frame True {
          n92 = call <vilib>:"Clear Errors.vi"("error in (no error)"=w400) -> ("error out"=w399:errorcluster)  [unwired: 5 in, 1 out]
        }
      }
    }
  }
  "error out" <- w2
